vi "注册.vi"() -> ()   [LabVIEW 2016]
panel:
  in  "路径":path
  out "注册状态":string
  in  "密  码":string
  in  "用户名":string
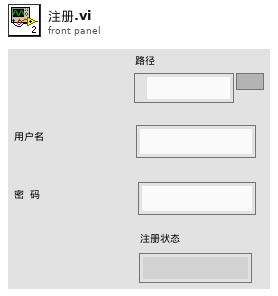
[diagram p1: front panel]
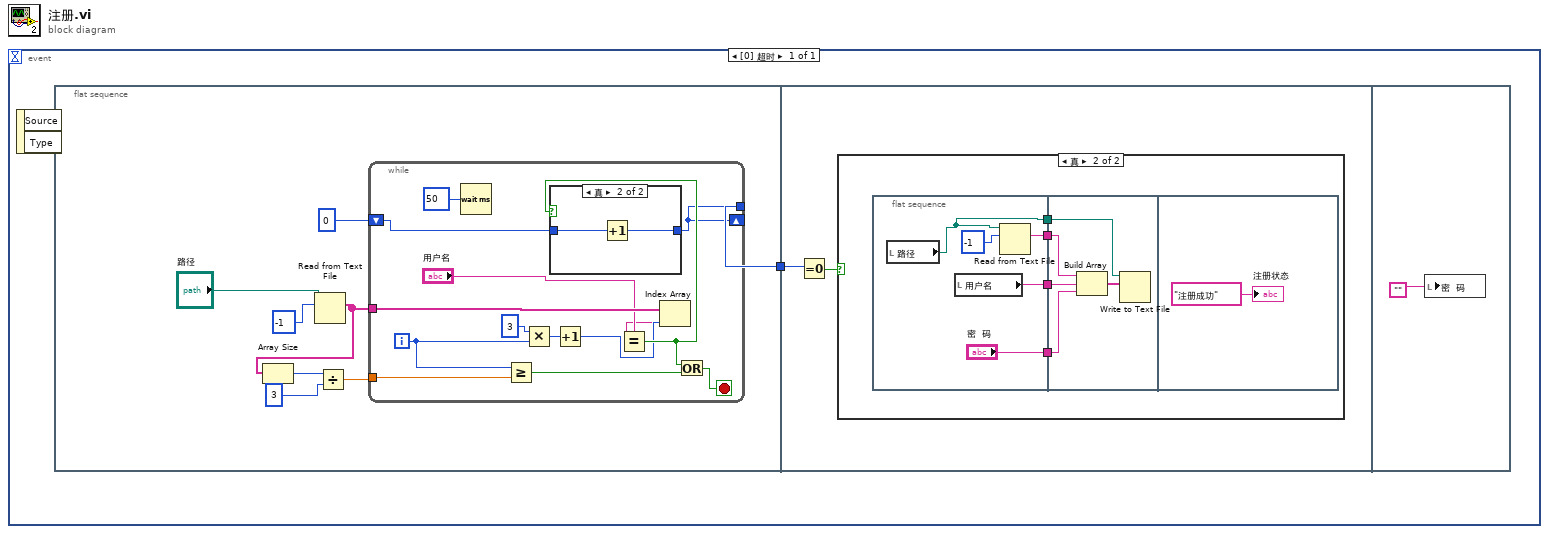
[diagram p0: block diagram]
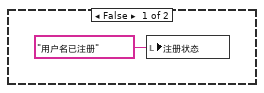
[diagram p3: hidden frame]
diagram:
  n1 = event shown="[0] 超时" {
    selector: _ -> [_]
    dyn-events: _ -> [_]
    timeout: _ -> [_]
    event Timeout {
      n2 = event-data() -> ()  [unwired: 1 in, 2 out]
      n3 = flat-sequence {
        tunnel: [w3] -> w1
        tunnel: w1 -> [w28]
        frame #0 {
          n4 = Read from Text File(file (use dialog)="路径", count=-1 ("计数")) -> (text=w6:string[])  [unwired: 2 in, 3 out]
          n5 = Array Size(array=w6) -> (size(s)=w8:i32)
          n6 = Divide(x=w8, y=3) -> (x/y=w4:dbl)
          n7 = while {
            tunnel: w6 -> [w23]
            shift-right: [w14] -> _
            shift-left: 0 -> [w20]
            tunnel: w4 -> [w18]
            tunnel: [w14] -> w3
            i -> [w12]
            stop <- w15 stop-if-true
            n8 = Wait (ms)(milliseconds to wait=u32 50 ("等待时间（毫秒）")) -> ()  [unwired: 1 out]
            n9 = Greater Or Equal?(x=w12, y=w18) -> (x >= y?=w16:bool)
            n10 = Multiply(x=3, y=w12) -> (x*y=w19:i32)
            n11 = Increment(x=w19) -> (x+1=w13:i32)
            n12 = Index Array(array=w23, index=w13) -> (element=w11:string)
            n13 = Equal?(x="用户名", y=w11) -> (x = y?=w17:bool)
            n14 = case shown="真" w17 {
              tunnel: w20 -> [w24 w26]
              tunnel: [w24 w25] -> w14
              frame False {
              }
              frame True {
                n15 = Increment(x=w26) -> (x+1=w25:i32)
              }
            }
            n16 = Or(x=w17, y=w16) -> (x .or. y?=w15:bool)
          }
        }
        frame #1 {
          n17 = Equal To 0?(x=w28) -> (x = 0?=w27:bool)
          n18 = case shown="真" w27 {
            frame False {
              n19 = local write "注册状态"("用户名已注册") -> ()
            }
            frame True {
              n20 = flat-sequence {
                tunnel: ["密  码"] -> w33
                tunnel: [w37] -> w32
                tunnel: [w35] -> w31
                tunnel: [w34] -> w30
                tunnel: w31 -> [w42]
                tunnel: w32 -> [w39]
                tunnel: w33 -> [w40]
                tunnel: w30 -> [w41]
                frame #0 {
                  n21 = local read "路径"() -> (w34:path)
                  n22 = local read "用户名"() -> (w37:string)
                  n23 = Read from Text File(file (use dialog)=w34, count=-1 ("计数")) -> (text=w35:string)  [unwired: 2 in, 3 out]
                }
                frame #1 {
                  n24 = Build Array(w42, w39, w40) -> (w43:string[])
                  n25 = Write to Text File(file (use dialog)=w41, text=w43) -> ()  [unwired: 2 in, 3 out]
                }
                frame #2 {
                  "注册状态" <- "注册成功"
                }
              }
            }
          }
        }
        frame #2 {
          n26 = local write "密  码"("") -> ()
        }
      }
    }
  }
